vi "String - Channel to Probe Mappings.vi"(6 "Channel to Probe Mapping":string, 8 "error in (no error)":errorcluster, 9 "Channel to Probe Cluster Label":string[](array[string]), 10 "ColHdrString":string[](array[string]), 11 "ItemNames":string[][](array[string])) -> (0 "error out":errorcluster, 1 "Probe List Valid":bool, 2 "Probe List":i32[](array[numeric]), 3 "Available Probe List":string, 4 "cRIO Channel List":i32[](array[numeric]), 5 "Duplicate":bool, 7 "Duplicated Probe #":i32)   [LabVIEW 2013]
panel:
  out "All rows have at least 1 Probe":bool
  out "# of Probes for each Row":i32[](array[numeric])
  out "Matched Probe List":i32[](array[numeric])
  out "Available Probe List":i32[](array[numeric])
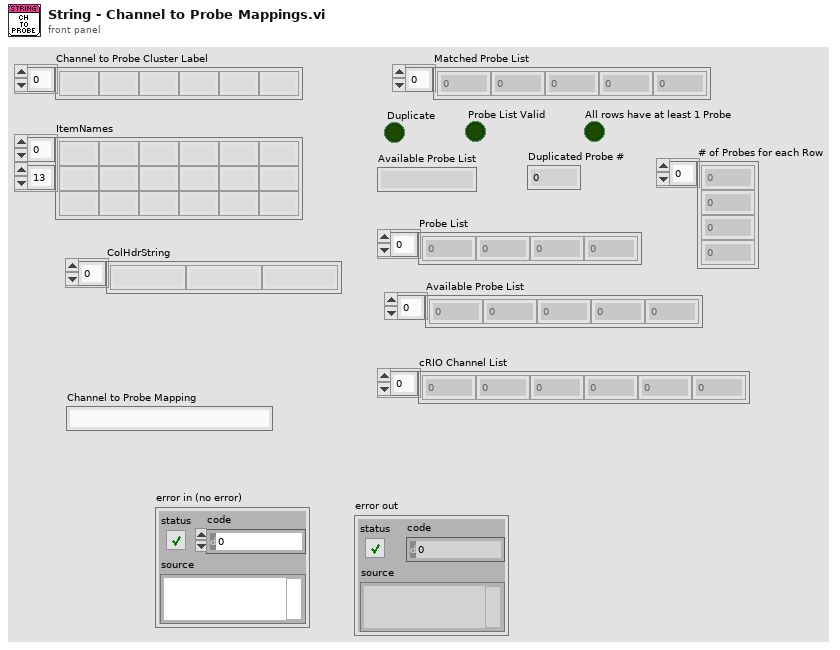
[diagram p1: front panel]
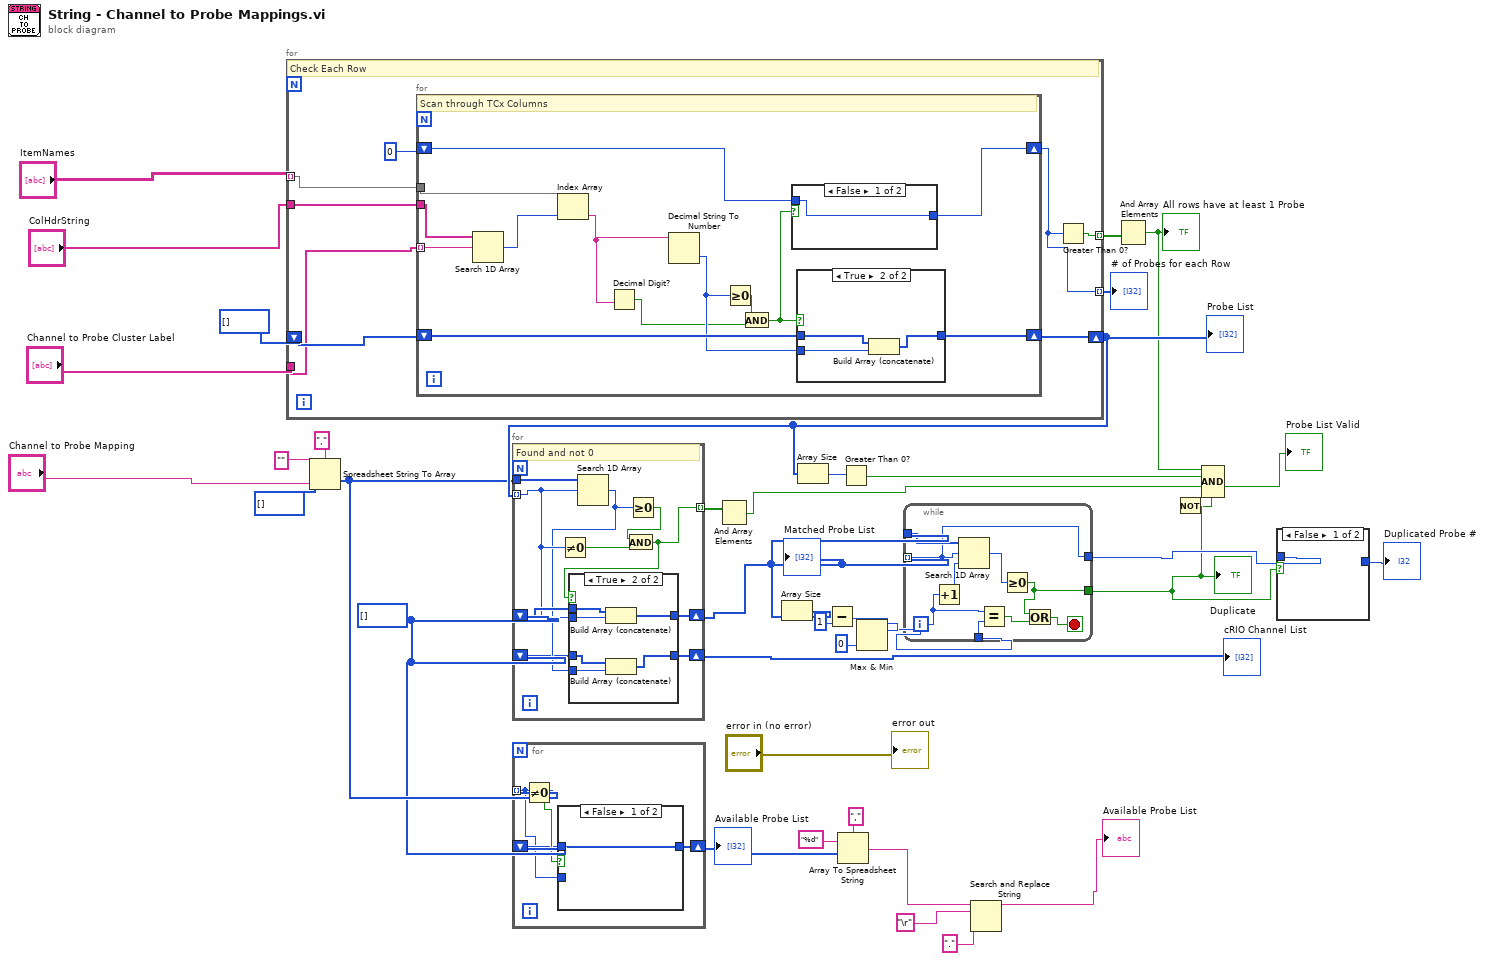
[diagram p0: block diagram]
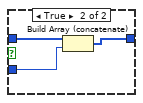
[diagram p3: hidden frame]
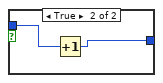
[diagram p5: hidden frame]
diagram:
  w19 = i32[] []
  n1 = for {
    tunnel: "ItemNames" -> [w46] mode=indexing
    tunnel: "ColHdrString" -> [w44]
    tunnel: "Channel to Probe Cluster Label" -> [w43]
    shift-right: [w42] -> w25
    shift-left: i32[] [] -> [w45]
    tunnel: [w39] -> w3 mode=indexing
    tunnel: [w41] -> w2 mode=indexing
    # "Check Each Row"
    n2 = for {
      tunnel: w46 -> [w59]
      shift-right: [w50] -> w42
      shift-left: w45 -> [w58]
      tunnel: w44 -> [w53]
      tunnel: w43 -> [w52] mode=indexing
      shift-right: [w48] -> w39
      shift-left: 0 -> [w47]
      # "Scan through TCx Columns"
      n3 = Search 1D Array(1D array=w53, element=w52) -> (index of element=w51:i32)  [unwired: 1 in]
      n4 = Index Array(array=w59, index=w51) -> (element=w55:string)
      n5 = Decimal Digit?(1:w55) -> (0:w54:bool)
      n6 = Decimal String To Number(string=w55) -> (number=w57:i32)  [unwired: 2 in, 1 out]
      n7 = Greater Or Equal To 0?(x=w57) -> (x >= 0?=w56:bool)
      n8 = And(x=w56, y=w54) -> (x .and. y?=w49:bool)
      n9 = case shown="False" w49 {
        tunnel: [w60 w62] -> w48
        tunnel: w47 -> [w60 w61]
        frame False {
        }
        frame True {
          n10 = Increment(x=w61) -> (x+1=w62:i32)
        }
      }
      n11 = case shown="True" w49 {
        tunnel: w57 -> [_ w66]
        tunnel: [w63 w65] -> w50
        tunnel: w58 -> [w63 w64]
        frame False {
        }
        frame True {
          n12 = Build Array (concatenate)(w64, w66) -> (w65:i32[])
        }
      }
    }
    n13 = Greater Than 0?(x=w39) -> (x > 0?=w41:bool)
  }
  "Probe List" <- w25
  "# of Probes for each Row" <- w3
  n14 = Spreadsheet String To Array(delimiter (Tab)=",", format string="", spreadsheet string="Channel to Probe Mapping", array type (2D Dbl)=i32[] []) -> (array=w20:i32[])
  n15 = for {
    tunnel: w25 -> [w72] mode=indexing
    tunnel: w20 -> [w76]
    tunnel: [w70] -> w33 mode=indexing
    shift-right: [w75] -> w17
    shift-left: w19 -> [w74]
    shift-right: [w67] -> w38
    shift-left: w19 -> [w68]
    # "Found and not 0"
    n16 = Not Equal To 0?(x=w72) -> (x != 0?=w71:bool)
    n17 = Search 1D Array(1D array=w76, element=w72) -> (index of element=w69:i32)  [unwired: 1 in]
    n18 = Greater Or Equal To 0?(x=w69) -> (x >= 0?=w73:bool)
    n19 = And(x=w73, y=w71) -> (x .and. y?=w70:bool)
    n20 = case shown="True" w70 {
      tunnel: w72 -> [_ w84]
      tunnel: [w78 w83] -> w75
      tunnel: w74 -> [w78 w82]
      tunnel: w69 -> [_ w81]
      tunnel: w68 -> [w77 w80]
      tunnel: [w77 w79] -> w67
      frame False {
      }
      frame True {
        n21 = Build Array (concatenate)(w82, w84) -> (w83:i32[])
        n22 = Build Array (concatenate)(w80, w81) -> (w79:i32[])
      }
    }
  }
  "cRIO Channel List" <- w38
  "Matched Probe List" <- w17
  n23 = for {
    tunnel: w20 -> [w86] mode=indexing
    shift-right: [w85] -> w18
    shift-left: w19 -> [w87]
    n24 = Not Equal To 0?(x=w86) -> (x != 0?=w88:bool)
    n25 = case shown="False" w88 {
      tunnel: w87 -> [w89 w92]
      tunnel: w86 -> [_ w91]
      tunnel: [w89 w90] -> w85
      frame False {
      }
      frame True {
        n26 = Build Array (concatenate)(w92, w91) -> (w90:i32[])
      }
    }
  }
  "Available Probe List" <- w18
  n27 = And Array Elements(Boolean array=w33) -> (logical AND=w22:bool)
  n28 = Array Size(array=w17) -> (size(s)=w16:i32)
  n29 = Array Size(array=w25) -> (size(s)=w24:i32)
  n30 = Subtract(x=w16, y=1) -> (x-y=w14:i32)
  n31 = Array To Spreadsheet String(delimiter (Tab)=",", array=w18, 3:"%d" ("format string")) -> (spreadsheet string=w7:string)
  n32 = Greater Than 0?(x=w24) -> (x > 0?=w23:bool)
  n33 = Max & Min(x=w14, y=0) -> (max(x,y)=w12:i32)  [unwired: 1 out]
  n34 = while {
    tunnel: w17 -> [w93] mode=indexing
    tunnel: w17 -> [w101]
    tunnel: w12 -> [w97]
    tunnel: [w94] -> w9
    tunnel: [w93] -> w11
    i -> [w98]
    stop <- w95 stop-if-true
    n35 = Increment(x=w98) -> (x+1=w100:i32)
    n36 = Search 1D Array(1D array=w101, element=w93, start index (0)=w100) -> (index of element=w99:i32)
    n37 = Equal?(x=w98, y=w97) -> (x = y?=w96:bool)
    n38 = Greater Or Equal To 0?(x=w99) -> (x >= 0?=w94:bool)
    n39 = Or(x=w94, y=w96) -> (x .or. y?=w95:bool)
  }
  "Duplicate" <- w9
  n40 = Search and Replace String(input string=w7, search string="\r", replace string="." ("replace string (\"\")")) -> (result string=→"Available Probe List":string)  [unwired: 5 in, 3 out]
  n41 = And Array Elements(Boolean array=w2) -> (logical AND=w1:bool)
  "All rows have at least 1 Probe" <- w1
  n42 = Not(x=w9) -> (.not. x?=w8:bool)
  n43 = Compound Arithmetic op=AND(w1, w23, w22, w8) -> (→"Probe List Valid":bool)
  n44 = case shown="False" w9 {
    tunnel: w11 -> [_ w102]
    tunnel: [_ w102] -> w10
    frame False {
    }
    frame True {
    }
  }
  "Duplicated Probe #" <- w10
  "error out" <- "error in (no error)"
